vi "Teleop.vi"() -> ()   [LabVIEW 2016]
doc: "This VI is called for each TeleOp packet received from the DS where the robot is not disabled. It is often used to read from the joysticks and update I/O or to update setpoints for timed control loops. It should complete and return within 20 milliseconds or it may miss DS packets."
uses:
  <vilib>/Rock Robotics/WPI/Utilities/WPI_GetSetVariantRefNum.vi
  External/2ndContollerStatus.vi
  External/External.lvlib
panel:
  out "Angle1":u16
  out "Angle0":u16
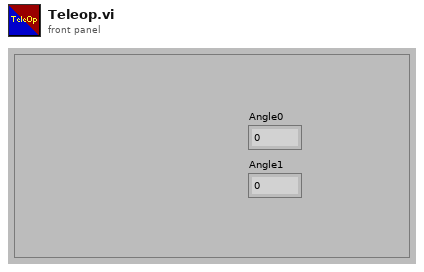
[diagram p1: front panel]
types:
  T1 = enum16{"A", "B", "X", "Y", "LB", "RB", "Back", "Start"}
  T2 = typedef "WPI_ServoDeviceRef.ctl" = cluster{"DeviceStatus":errorcluster, "PWM Channel":T3, "DeadBand":T4}
  T3 = typedef "FPGA_DIOPWMChannel.ctl" = enum8{"PWM 0", "PWM 1", "PWM 2", "PWM 3", "PWM 4", "PWM 5", "PWM 6", "PWM 7", "PWM 8", "PWM 9", "PWM MXP 0", "PWM MXP 1", "PWM MXP 2", "PWM MXP 3", "PWM MXP 4", "PWM MXP 5", "PWM MXP 6", "PWM MXP 7", "PWM MXP 8", "PWM MXP 9", "Invalid"}
  T4 = typedef "WPI_PWMDeadband.ctl" = cluster{"Name":string, "maxPositivePwm":i32, "minPositivePwm":i32, "centerPwm":i32, "maxNegativePwm":i32, "minNegativePwm":i32, "angularRange":u16}
  T5 = typedef "WPI_JoystickDevRef.ctl" = cluster{"Device":T6}
  T6 = typedef "WPI_JoystickDeviceEnum.ctl" = enum16{"USB 0", "USB 1", "USB 2", "USB 3", "USB 4", "USB 5"}
  T7 = typedef "WPI_RobotDriveDevRef.ctl" = cluster{"DevStatus":errorcluster, "Motors[]":T8[], "Square Inputs":bool, "Max Output":dbl}
  T8 = typedef "WPI_MotorControlDeviceRef.ctl" = cluster{"DeviceStatus":errorcluster, "Type":T9, "PWM":cluster{"PWM Channel":T3, "DeadBand":T4}, "CAN":cluster{"Device Number":u8, "SetOutput VI Ref":variant, "GetOutput VI Ref":variant, "Enable VI Ref":variant, "Disable VI Ref":variant, "Data":variant}, "Invert":bool}
  T9 = typedef "WPI_MotorControlType.ctl" = enum16{"PWM", "CAN"}
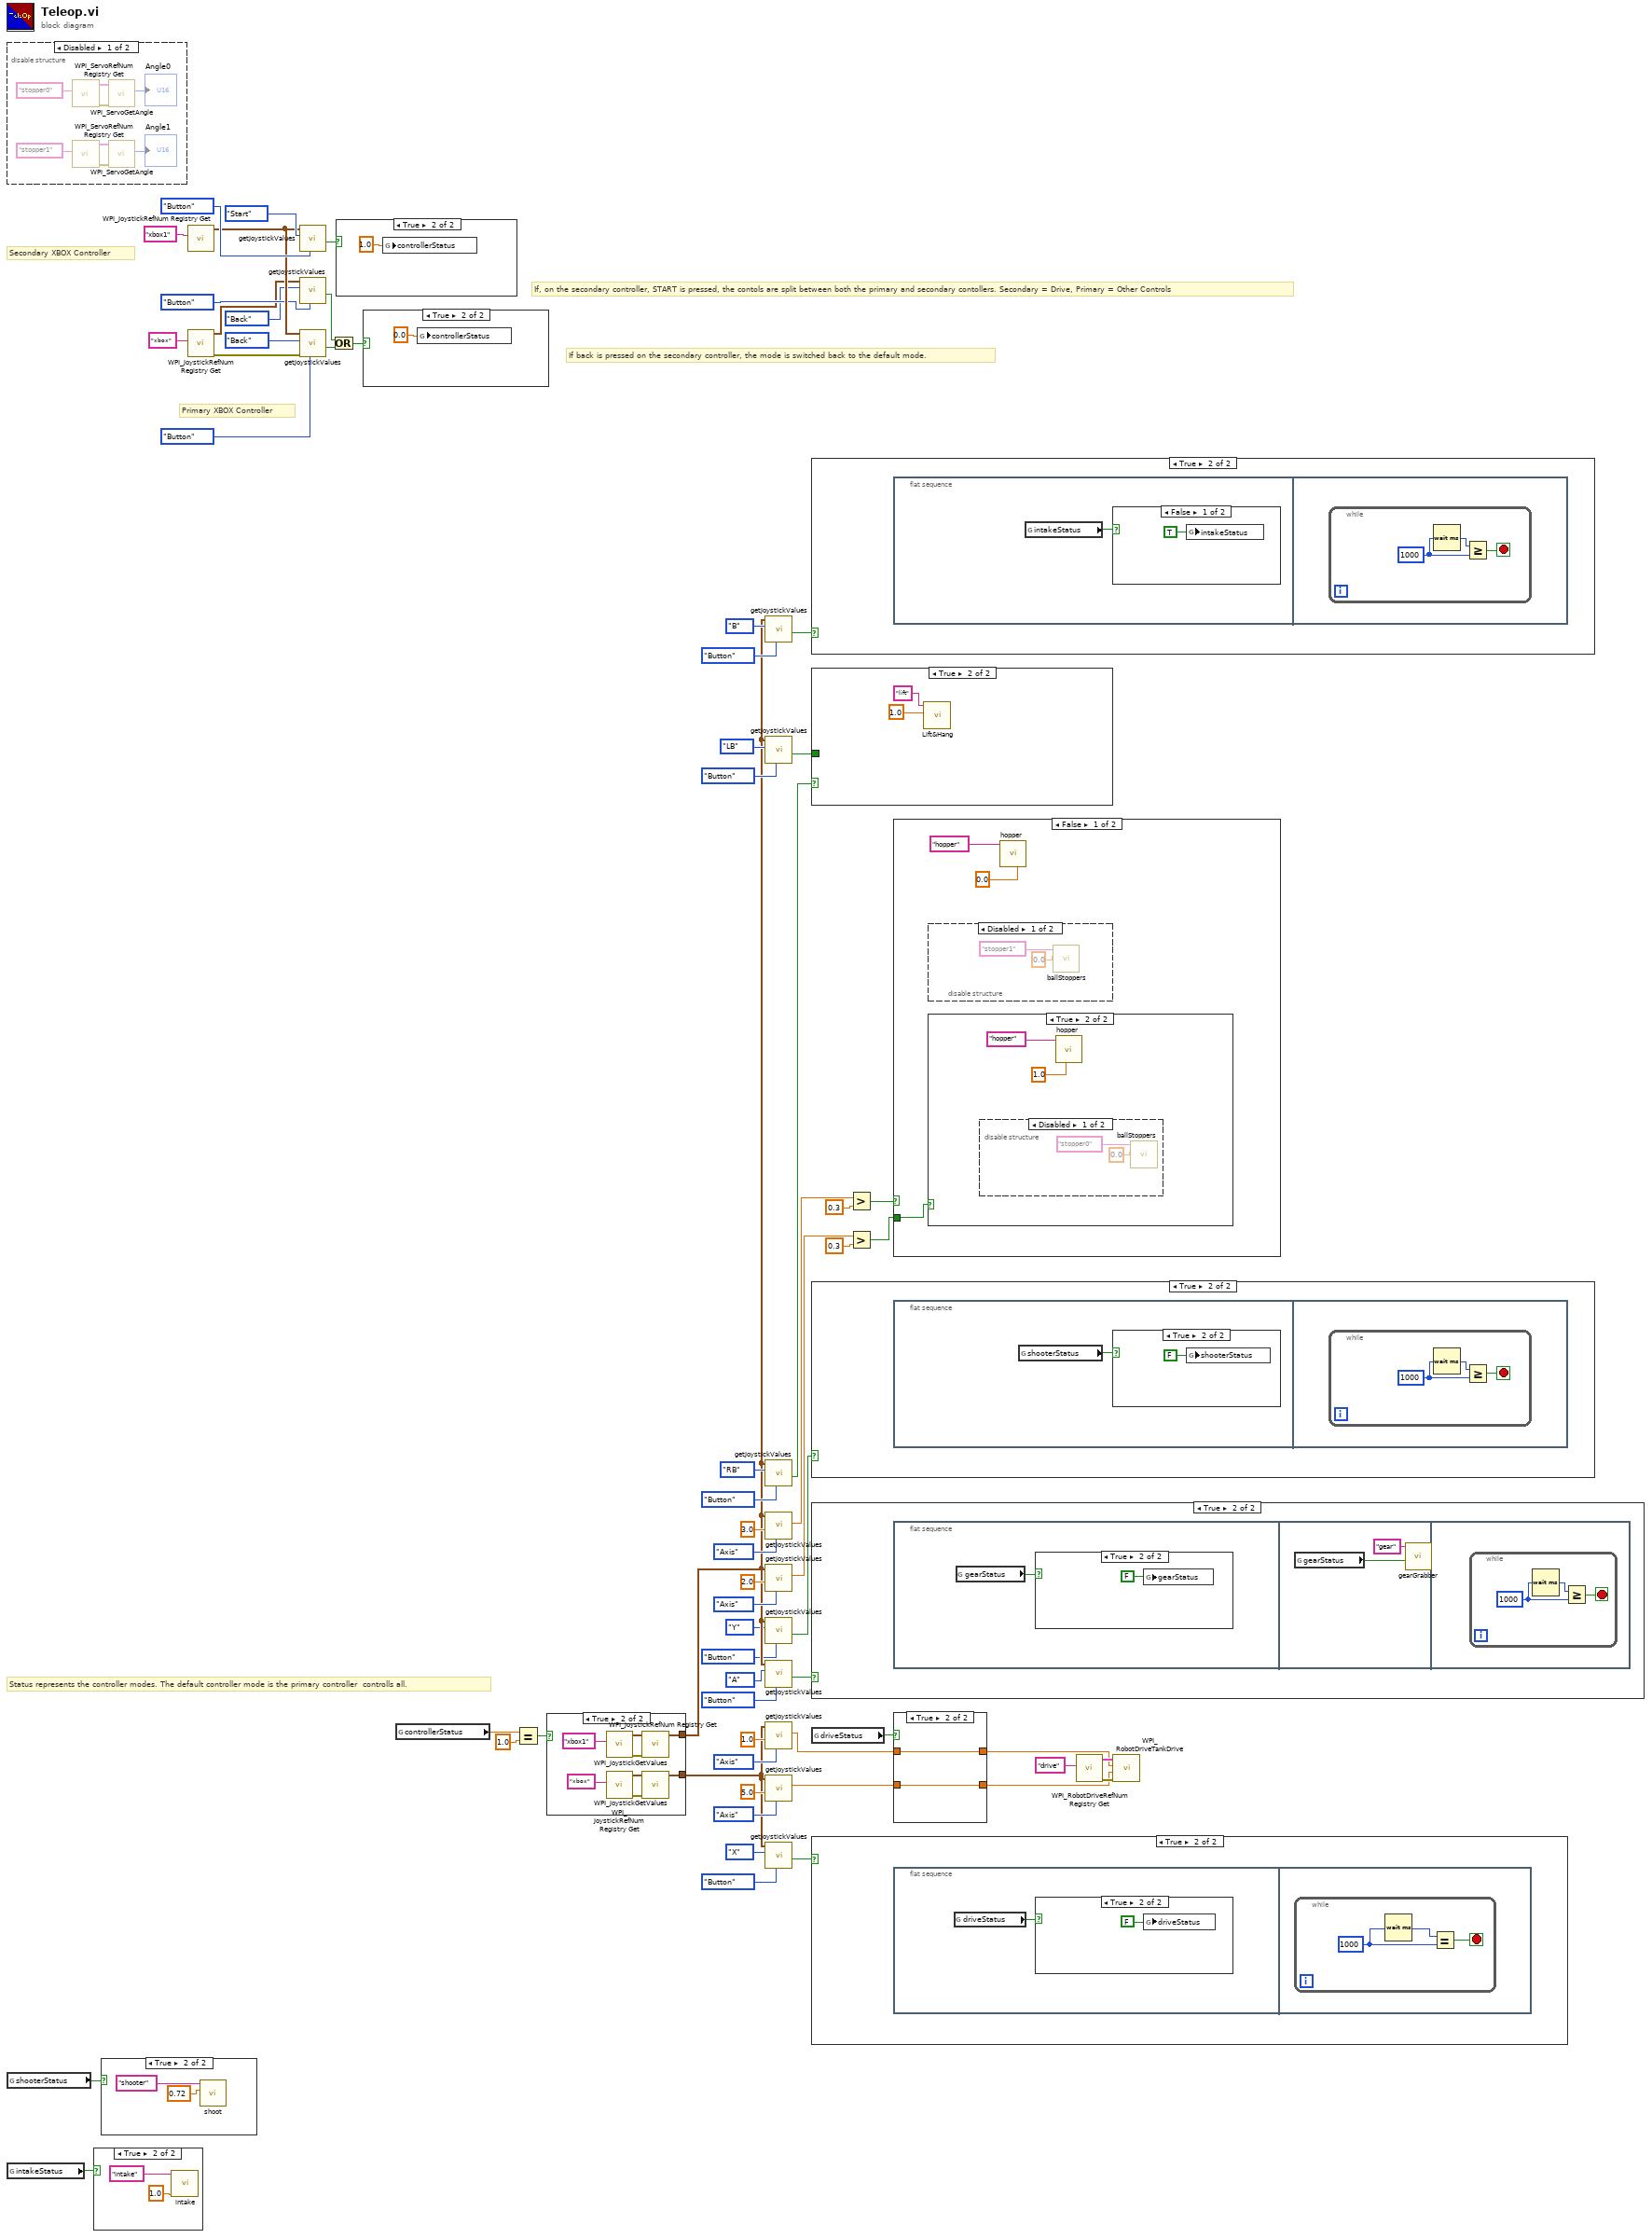
[diagram p0: block diagram]
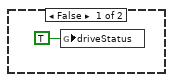
[diagram p3: hidden frame]
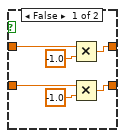
[diagram p4: hidden frame]
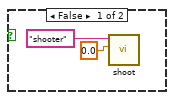
[diagram p5: hidden frame]
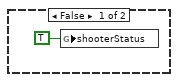
[diagram p7: hidden frame]
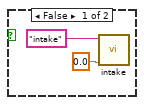
[diagram p8: hidden frame]
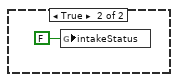
[diagram p11: hidden frame]
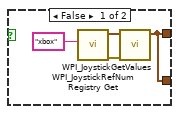
[diagram p12: hidden frame]
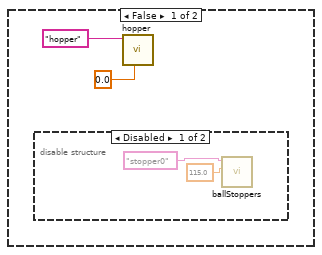
[diagram p14: hidden frame]
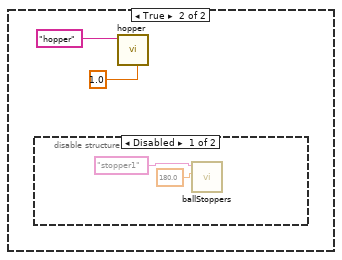
[diagram p17: hidden frame]
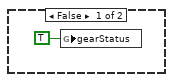
[diagram p20: hidden frame]
diagram:
  # "Status represents the controller modes. The default controller mode is the primary controller  controlls all."
  # "Secondary XBOX Controller"
  # "Primary XBOX Controller"
  # "If back is pressed on the secondary controller, the mode is switched back to the default mode."
  # "If, on the secondary controller, START is pressed, the contols are split between both the primary and secondary contollers. Secondary = Drive, Primary = Other Controls"
  n1 = disable-structure shown="Disabled" {
    frame Disabled {
      n2 = call <vilib>:"WPI_ServoRefNum Registry Get.vi"("refnum name"="stopper0") -> ("error out"=w64:errorcluster, "ServoDeviceRef"=w63:T2)  [unwired: 9 in]
      n3 = call <vilib>:"WPI_ServoRefNum Registry Get.vi"("refnum name"="stopper1") -> ("error out"=w68:errorcluster, "ServoDeviceRef"=w67:T2)  [unwired: 9 in]
      n4 = call <vilib>:"WPI_ServoGetAngle.vi"("ServoDeviceRef"=w63, "error in (no error)"=w64) -> ("Angle"=→"Angle0":u16)  [unwired: 6 in, 2 out]
      n5 = call <vilib>:"WPI_ServoGetAngle.vi"("ServoDeviceRef"=w67, "error in (no error)"=w68) -> ("Angle"=→"Angle1":u16)  [unwired: 6 in, 2 out]
    }
    frame Enabled {
    }
  }
  n6 = global read "2ndContollerStatus.vi" "shooterStatus"() -> (w10:bool)
  n7 = global read "2ndContollerStatus.vi" "intakeStatus"() -> (w15:bool)
  n8 = case shown="True" w15 {
    frame False {
      n9 = call "intake.vi"("intakeSpeed"=0.0, "intake"="intake") -> ()  [unwired: 9 in, 1 out]
    }
    frame True {
      n10 = call "intake.vi"("intakeSpeed"=1.0, "intake"="intake") -> ()  [unwired: 9 in, 1 out]
    }
  }
  n11 = case shown="True" w10 {
    frame False {
      n12 = call "shoot.vi"("Motor Power"=0.0, "refnum name"="shooter") -> ()  [unwired: 9 in, 1 out]
    }
    frame True {
      n13 = call "shoot.vi"("Motor Power"=0.72, "refnum name"="shooter") -> ()  [unwired: 9 in, 1 out]
    }
  }
  n14 = call <vilib>:"WPI_JoystickRefNum Registry Get.vi"("refnum name"="xbox1" ("xbox1")) -> ("JoystickDevRef"=w57:T5)  [unwired: 9 in, 1 out]
  n15 = call <vilib>:"WPI_JoystickRefNum Registry Get.vi"("refnum name"="xbox" ("xbox")) -> ("error out"=w56:errorcluster, "JoystickDevRef"=w49:T5)  [unwired: 9 in]
  n16 = call "getJoystickValues.vi"("Mode"=enum16{"Axis", "Button"}."Button", "buttonType"=T1."Start", "JoystickDevRef"=w57) -> ("Button Pressed"=w52:bool)  [unwired: 5 in, 3 out]
  n17 = call "getJoystickValues.vi"("Mode"=enum16{"Axis", "Button"}."Button", "buttonType"=T1."Back", "JoystickDevRef"=w49) -> ("Button Pressed"=w50:bool)  [unwired: 5 in, 3 out]
  n18 = call "getJoystickValues.vi"("Mode"=enum16{"Axis", "Button"}."Button", "error in (no error)"=w56, "buttonType"=T1."Back", "JoystickDevRef"=w57) -> ("Button Pressed"=w51:bool)  [unwired: 4 in, 3 out]
  n19 = Or(x=w50, y=w51) -> (x .or. y?=w48:bool)
  n20 = case shown="True" w52 {
    frame False {
    }
    frame True {
      n21 = global write "2ndContollerStatus.vi" "controllerStatus"(1.0 ("status")) -> ()
    }
  }
  n22 = case shown="True" w48 {
    frame False {
    }
    frame True {
      n23 = global write "2ndContollerStatus.vi" "controllerStatus"(0.0 ("status")) -> ()
    }
  }
  n24 = global read "2ndContollerStatus.vi" "controllerStatus"() -> (w23:dbl)
  n25 = Equal?(x=w23, y=1.0) -> (x = y?=w21:bool)
  n26 = case shown="True" w21 {
    tunnel: [w81 w89] -> w5
    tunnel: [w81 w85] -> w14
    frame False {
      n27 = call <vilib>:"WPI_JoystickRefNum Registry Get.vi"("refnum name"="xbox") -> ("error out"=w83:errorcluster, "JoystickDevRef"=w82:T5)  [unwired: 9 in]
      n28 = call <vilib>:"WPI_JoystickGetValues.vi"("error in (no error)"=w83, "JoystickDevRef"=w82) -> ("JoystickDevRef"=w81:T5)  [unwired: 5 in, 4 out]
    }
    frame True {
      n29 = call <vilib>:"WPI_JoystickRefNum Registry Get.vi"("refnum name"="xbox1") -> ("error out"=w87:errorcluster, "JoystickDevRef"=w86:T5)  [unwired: 9 in]
      n30 = call <vilib>:"WPI_JoystickRefNum Registry Get.vi"("refnum name"="xbox") -> ("error out"=w91:errorcluster, "JoystickDevRef"=w90:T5)  [unwired: 9 in]
      n31 = call <vilib>:"WPI_JoystickGetValues.vi"("error in (no error)"=w87, "JoystickDevRef"=w86) -> ("JoystickDevRef"=w85:T5)  [unwired: 5 in, 4 out]
      n32 = call <vilib>:"WPI_JoystickGetValues.vi"("error in (no error)"=w91, "JoystickDevRef"=w90) -> ("JoystickDevRef"=w89:T5)  [unwired: 5 in, 4 out]
    }
  }
  n33 = call "getJoystickValues.vi"("Mode"=enum16{"Axis", "Button"}."Button", "buttonType"=T1."B", "JoystickDevRef"=w14) -> ("Button Pressed"=w16:bool)  [unwired: 5 in, 3 out]
  n34 = call "getJoystickValues.vi"("Mode"=enum16{"Axis", "Button"}."Button", "buttonType"=T1."LB", "JoystickDevRef"=w14) -> ("Button Pressed"=w38:bool)  [unwired: 5 in, 3 out]
  n35 = call "getJoystickValues.vi"("Mode"=enum16{"Axis", "Button"}."Button", "buttonType"=T1."RB", "JoystickDevRef"=w14) -> ("Button Pressed"=w43:bool)  [unwired: 5 in, 3 out]
  n36 = call "getJoystickValues.vi"("Mode"=enum16{"Axis", "Button"}."Axis", "Axis"=3.0, "JoystickDevRef"=w14) -> ("Value"=w25:dbl)  [unwired: 5 in, 3 out]
  n37 = call "getJoystickValues.vi"("Mode"=enum16{"Axis", "Button"}."Axis", "Axis"=2.0, "JoystickDevRef"=w14) -> ("Value"=w24:dbl)  [unwired: 5 in, 3 out]
  n38 = call "getJoystickValues.vi"("Mode"=enum16{"Axis", "Button"}."Button", "buttonType"=T1."Y", "JoystickDevRef"=w14) -> ("Button Pressed"=w11:bool)  [unwired: 5 in, 3 out]
  n39 = call "getJoystickValues.vi"("Mode"=enum16{"Axis", "Button"}."Button", "buttonType"=T1."A", "JoystickDevRef"=w14) -> ("Button Pressed"=w34:bool)  [unwired: 5 in, 3 out]
  n40 = call "getJoystickValues.vi"("Mode"=enum16{"Axis", "Button"}."Axis", "Axis"=1.0, "JoystickDevRef"=w5) -> ("Value"=w8:dbl)  [unwired: 5 in, 3 out]
  n41 = call "getJoystickValues.vi"("Mode"=enum16{"Axis", "Button"}."Axis", "Axis"=5.0, "JoystickDevRef"=w5) -> ("Value"=w6:dbl)  [unwired: 5 in, 3 out]
  n42 = call "getJoystickValues.vi"("Mode"=enum16{"Axis", "Button"}."Button", "buttonType"=T1."X", "JoystickDevRef"=w5) -> ("Button Pressed"=w2:bool)  [unwired: 5 in, 3 out]
  n43 = case shown="True" w16 {
    frame False {
    }
    frame True {
      n44 = flat-sequence {
        frame #0 {
          n45 = global read "2ndContollerStatus.vi" "intakeStatus"() -> (w93:bool)
          n46 = case shown="False" w93 {
            frame False {
              n47 = global write "2ndContollerStatus.vi" "intakeStatus"(TRUE ("intakeStatus")) -> ()
            }
            frame True {
              n48 = global write "2ndContollerStatus.vi" "intakeStatus"(FALSE ("intakeStatus")) -> ()
            }
          }
        }
        frame #1 {
          n49 = while {
            stop <- w96 stop-if-true
            w98 = u32 1000 ("milliseconds to wait")
            n50 = Wait (ms)(milliseconds to wait=w98) -> (millisecond timer value=w97:u32)
            n51 = Greater Or Equal?(x=w97, y=w98) -> (x >= y?=w96:bool)
          }
        }
      }
    }
  }
  n52 = case shown="True" w43 {
    tunnel: w38 -> [w99 _]
    frame False {
      n53 = case shown="False" w99 {
        frame False {
          n54 = call "Lift&Hang.vi"("status"=0.0, "refnum name"="lift" ("lift")) -> ()  [unwired: 9 in, 1 out]
        }
        frame True {
          n55 = call "Lift&Hang.vi"("status"=-1.0, "refnum name"="lift" ("lift")) -> ()  [unwired: 9 in, 1 out]
        }
      }
    }
    frame True {
      n56 = call "Lift&Hang.vi"("status"=1.0, "refnum name"="lift" ("lift")) -> ()  [unwired: 9 in, 1 out]
    }
  }
  n57 = case shown="True" w11 {
    frame False {
    }
    frame True {
      n58 = flat-sequence {
        frame #0 {
          n59 = global read "2ndContollerStatus.vi" "shooterStatus"() -> (w106:bool)
          n60 = case shown="True" w106 {
            frame False {
              n61 = global write "2ndContollerStatus.vi" "shooterStatus"(TRUE ("shooterStatus")) -> ()
            }
            frame True {
              n62 = global write "2ndContollerStatus.vi" "shooterStatus"(FALSE ("shooterStatus")) -> ()
            }
          }
        }
        frame #1 {
          n63 = while {
            stop <- w109 stop-if-true
            w111 = u32 1000 ("milliseconds to wait")
            n64 = Wait (ms)(milliseconds to wait=w111) -> (millisecond timer value=w110:u32)
            n65 = Greater Or Equal?(x=w110, y=w111) -> (x >= y?=w109:bool)
          }
        }
      }
    }
  }
  n66 = case shown="True" w34 {
    frame False {
    }
    frame True {
      n67 = flat-sequence {
        frame #0 {
          n68 = global read "2ndContollerStatus.vi" "gearStatus"() -> (w112:bool)
          n69 = case shown="True" w112 {
            frame False {
              n70 = global write "2ndContollerStatus.vi" "gearStatus"(TRUE ("gearStatus")) -> ()
            }
            frame True {
              n71 = global write "2ndContollerStatus.vi" "gearStatus"(FALSE ("gearStatus")) -> ()
            }
          }
        }
        frame #1 {
          n72 = global read "2ndContollerStatus.vi" "gearStatus"() -> (w115:bool)
          n73 = call "gearGrabber.vi"("gearStatus"=w115, "gear"="gear") -> ()  [unwired: 9 in, 1 out]
        }
        frame #2 {
          n74 = while {
            stop <- w119 stop-if-true
            w117 = u32 1000 ("milliseconds to wait")
            n75 = Wait (ms)(milliseconds to wait=w117) -> (millisecond timer value=w118:u32)
            n76 = Greater Or Equal?(x=w118, y=w117) -> (x >= y?=w119:bool)
          }
        }
      }
    }
  }
  n77 = global read "2ndContollerStatus.vi" "driveStatus"() -> (w1:bool)
  n78 = case shown="True" w2 {
    frame False {
    }
    frame True {
      n79 = flat-sequence {
        frame #0 {
          n80 = global read "2ndContollerStatus.vi" "driveStatus"() -> (w120:bool)
          n81 = case shown="True" w120 {
            frame False {
              n82 = global write "2ndContollerStatus.vi" "driveStatus"(TRUE ("driveStatus")) -> ()
            }
            frame True {
              n83 = global write "2ndContollerStatus.vi" "driveStatus"(FALSE ("driveStatus")) -> ()
            }
          }
        }
        frame #1 {
          n84 = while {
            stop <- w123 stop-if-true
            w124 = u32 1000 ("milliseconds to wait")
            n85 = Wait (ms)(milliseconds to wait=w124) -> (millisecond timer value=w125:u32)
            n86 = Equal?(x=w125, y=w124) -> (x = y?=w123:bool)
          }
        }
      }
    }
  }
  n87 = Greater?(x=w25, y=0.3) -> (0:w27:bool)
  n88 = Greater?(x=w24, y=0.3) -> (0:w26:bool)
  n89 = case shown="False" w27 {
    tunnel: w26 -> [w128 _]
    frame False {
      n90 = disable-structure shown="Disabled" {
        frame Disabled {
          n91 = call "ballStoppers.vi"("stopperValue"=0.0, "stopper1 or stopper0"="stopper1") -> ()  [unwired: 9 in, 1 out]
        }
        frame Enabled {
        }
      }
      n92 = case shown="True" w128 {
        frame False {
          n93 = disable-structure shown="Disabled" {
            frame Disabled {
              n94 = call "ballStoppers.vi"("stopperValue"=115.0, "stopper1 or stopper0"="stopper0") -> ()  [unwired: 9 in, 1 out]
            }
            frame Enabled {
            }
          }
          n95 = call "hopper.vi"("Left axis value"=0.0 ("Right axis value"), "hopper"="hopper") -> ()  [unwired: 9 in, 1 out]
        }
        frame True {
          n96 = disable-structure shown="Disabled" {
            frame Disabled {
              n97 = call "ballStoppers.vi"("stopperValue"=0.0, "stopper1 or stopper0"="stopper0") -> ()  [unwired: 9 in, 1 out]
            }
            frame Enabled {
            }
          }
          n98 = call "hopper.vi"("Left axis value"=1.0, "hopper"="hopper") -> ()  [unwired: 9 in, 1 out]
        }
      }
      n99 = call "hopper.vi"("Right axis value"=0.0, "hopper"="hopper") -> ()  [unwired: 9 in, 1 out]
    }
    frame True {
      n100 = disable-structure shown="Disabled" {
        frame Disabled {
          n101 = call "ballStoppers.vi"("stopperValue"=180.0, "stopper1 or stopper0"="stopper1") -> ()  [unwired: 9 in, 1 out]
        }
        frame Enabled {
        }
      }
      n102 = call "hopper.vi"("Right axis value"=1.0, "hopper"="hopper") -> ()  [unwired: 9 in, 1 out]
    }
  }
  n103 = case shown="True" w1 {
    tunnel: [w146 w150] -> w9
    tunnel: w8 -> [w148 w150]
    tunnel: [w144 w149] -> w7
    tunnel: w6 -> [w145 w149]
    frame False {
      n104 = Multiply(x=w148, y=-1.0) -> (x*y=w146:dbl)
      n105 = Multiply(x=w145, y=-1.0) -> (x*y=w144:dbl)
    }
    frame True {
    }
  }
  n106 = call <vilib>:"WPI_RobotDriveRefNum Registry Get.vi"("refnum name"="drive") -> ("error out"=w36:errorcluster, "RobotDriveDevRef"=w37:T7)  [unwired: 9 in]
  n107 = call <vilib>:"WPI_RobotDriveTankDrive.vi"("error in (no error)"=w36, "Right axis value"=w7, "Left axis value"=w9, "RobotDriveDevRef"=w37) -> ()  [unwired: 5 in, 3 out]
